vi "Get RFmx VNA Session.vi"(0 "TSM Context":T1, 5 "Pin":string, 11 "error in":errorcluster) -> (4 "RFmx VNA Session":refnum<k21>, 6 "Port":string, 15 "error out":errorcluster)   [LabVIEW 2023, in "RFCalAndFixtureCharact.Common.lvlib"]
uses:
  <vilib>/NI_TestStand_SemiconductorModule/NI_TestStand_Semiconductor_Module.lvlibp/PinMap/General/SemiconductorModuleContext.ctl
  Global Data Id Prefix.vi
  RFCalAndFixtureCharact.Common.lvlib
  <vilib>/NI_TestStand_SemiconductorModule/NI_TestStand_Semiconductor_Module.lvlibp
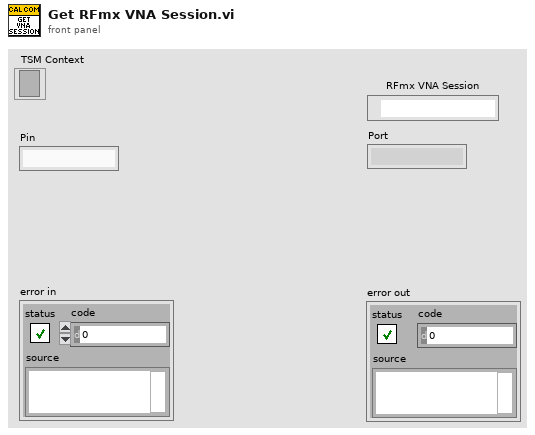
[diagram p1: front panel]
types:
  T1 = typedef "NI_TestStand_Semiconductor_Module.lvlibp/SemiconductorModuleContext.ctl" = refnum<k7>
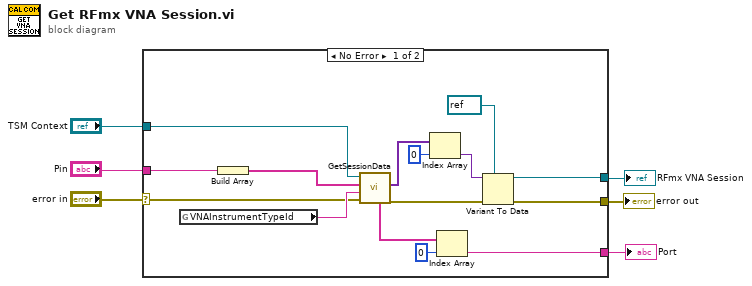
[diagram p0: block diagram]
diagram:
  n1 = case shown="No Error" "error in" {
    selector: "error in" -> [w19 w22]
    tunnel: "TSM Context" -> [w21 _]
    tunnel: [w12 w22] -> w5
    tunnel: "Pin" -> [w18 _]
    tunnel: [w11 _] -> w1
    tunnel: [w8 _] -> w2
    frame No Error {
      n2 = global read "Global Data Id Prefix.vi" "VNAInstrumentTypeId"() -> (w20:string)
      n3 = Build Array(w18) -> (w17:string[])
      n4 = call <vilib>:"GetSessionData.vi"("error in (no error)"=w19, "Instrument Type Id"=w20, "Pins"=w17, "Semiconductor Module Context"=w21) -> ("error out"=w13:errorcluster, "Session Data"=w16:variant[], "Channel Lists"=w10:string[])  [unwired: 2 in, 3 out]
      n5 = Index Array(array=w16, index=0) -> (element=w14:variant)
      n6 = Index Array(array=w10, index=0) -> (element=w8:string)
      n7 = Variant To Data(error in=w13, type=refnum<k21> refnum ("RFmx VNA Session 2"), Variant=w14) -> (data=w11:refnum<k21>, error out=w12:errorcluster)
    }
    frame Error {
    }
  }
  "error out" <- w5
  "Port" <- w2
  "RFmx VNA Session" <- w1
